vi "convert_from_json.vi"(8 "error in (no error)":errorcluster, 11 "json_path":path) -> (0 "error out":errorcluster, 3 "data_set":variant)   [LabVIEW 2015, in "lv-unit-conversion.lvlib"]
uses:
  lv-unit-conversion.lvlib
  _controls/data_set.ctl
  _controls/unit_set.ctl
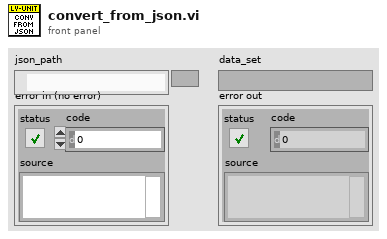
[diagram p1: front panel]
types:
  T1 = typedef "lv-unit-conversion.lvlib/data_set.ctl" = cluster{"unit_set":T2[]}
  T2 = typedef "lv-unit-conversion.lvlib/unit_set.ctl" = cluster{"symbol":string, "name":string, "dimension":string, "is_si_unit":bool, "category":string, "base_unit":string, "conversion_reference":string, "is_exact":bool, "a":dbl, "b":dbl, "c":dbl, "d":dbl, "underlying_def":string, "description":string}
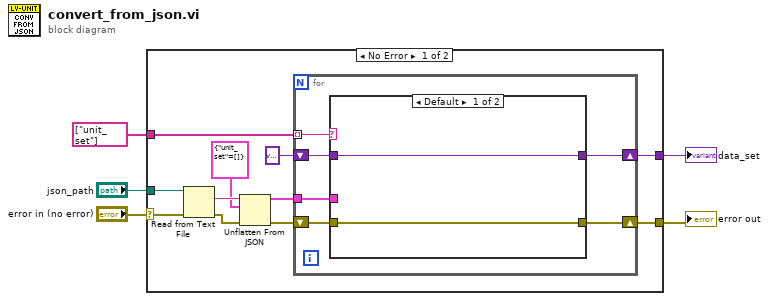
[diagram p0: block diagram]
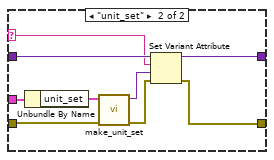
[diagram p2: hidden frame]
diagram:
  n1 = case shown="No Error" "error in (no error)" {
    selector: "error in (no error)" -> [w15 w34]
    tunnel: string[] ["unit_set"] -> [w10 _]
    tunnel: [w6 w34] -> w3
    tunnel: "json_path" -> [w16 _]
    tunnel: [w8 _] -> w1
    frame No Error {
      n2 = Read from Text File(file (use dialog)=w16, error in=w15) -> (text=w14:string, error out=w12:errorcluster)  [unwired: 2 in, 2 out]
      n3 = Unflatten From JSON(JSON string=w14, type and defaults=T1 {"unit_set"=[]} ("data_set"), error in (no error)=w12) -> (value=w11:T1, error out=w7:errorcluster)  [unwired: 4 in]
      n4 = for {
        tunnel: w11 -> [w21]
        tunnel: w10 -> [w22] mode=indexing
        shift-right: [w20] -> w8
        shift-left: variant -> [w19]
        shift-right: [w17] -> w6
        shift-left: w7 -> [w18]
        n5 = case shown="Default" w22 {
          selector: w22 -> [_ w28]
          tunnel: w21 -> [_ w33]
          tunnel: [w24 w29] -> w20
          tunnel: w19 -> [w24 w30]
          tunnel: w18 -> [w23 w31]
          tunnel: [w23 w25] -> w17
          frame Default {
          }
          frame "unit_set" {
            n6 = Unbundle By Name(w33) -> ("unit_set"=w32:T2[])
            n7 = call "make_unit_set.vi"("error in (no error)"=w31, "units []"=w32) -> ("error out"=w27:errorcluster, "unit_set out"=w26:variant)  [unwired: 8 in]
            n8 = Set Variant Attribute(Variant=w30, name=w28, value=w26, error in=w27) -> (Variant out=w29:variant, error out=w25:errorcluster)  [unwired: 1 out]
          }
        }
      }
    }
    frame Error {
    }
  }
  "error out" <- w3
  "data_set" <- w1
